vi "sub_DL950_main.vi"(8 "error in":errorcluster) -> (0 "error out":errorcluster, 3 "DL950 wfm":waveform(dbl)[](graph))   [LabVIEW 2019]
uses:
  _ctrl/create-rw-close.ctl
  _ctrl/fgv_DL950.ctl
  _ctrl/rw.ctl
  SubVIs/common/_ctrl/system-status.ctl
  SubVIs/common/Glob_Ref.vi
  Durability/common/Global 1.vi
panel:
  out "items":dbl[][](array[numeric])
  out "Data":string
  out "Waveform":cluster{"l":dbl, "dt":dbl, "Y":dbl[][]}(graph)
  out "n":i32
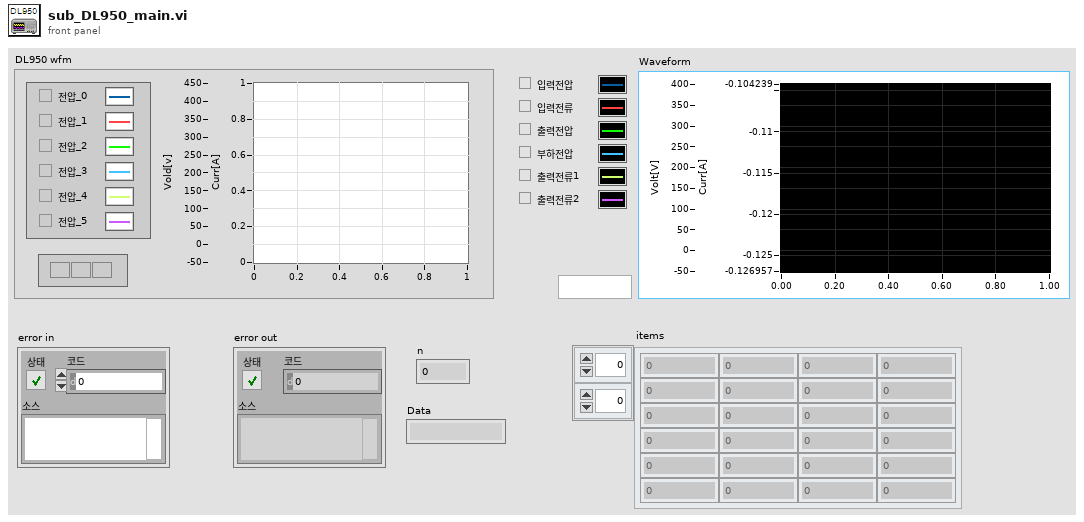
[diagram p1: front panel]
types:
  T1 = typedef "create-rw-close.ctl" = enum16{"create", "write", "read", "delete", "close"}
  T2 = typedef "fgv_DL950.ctl" = enum16{"init", "config", "Set-NCh", "setapply", "trigger", "history_clear", "read", "time-div", "wave-aquis", "start", "query", "abort", "set_items", "reset_items", "read_items", "percent_rise", "trigger_single", "stop", "offset cancel", "close"}
  T3 = typedef "rw.ctl" = enum16{"read", "write"}
  T4 = typedef "system-status.ctl" = enum16{"Initial", "Update", "Clear", "Read"}
  T5 = typedef "start.ctl" = enum16{"init", "open", "set", "start", "stop", "read", "read_items", "query", "close", "T_single", "reset", "exit"}
  T6 = typedef "DL950_wfms.ctl" = cluster{"wfms":waveform(dbl)[], "Waveform_2":cluster{"t0":dbl, "dt":dbl, "Y":dbl[][]}, "items":dbl[][], "da950_array":dbl[]}
  T7 = typedef "ref_all.ctl" = cluster{"BP4610 Config":refnum<vi>, "DSP1950 Config":refnum<vi>, "2470-config":refnum<vi>, "cDAQ 9269 AO config":refnum<vi>, "cDAQ 9221 Config":refnum<vi>, "cDAQ-9467 Config":refnum<vi>, "Waveform":refnum<vi>, "DL950 wfm":refnum<vi>, "AI Graph":refnum<vi>, "AO_Wave-config":refnum<vi>, "DL950 items":refnum<vi>, "Volt":refnum<vi>, "Current":refnum<vi>, "AO_Level":refnum<vi>, "RC-Test Judgement ":refnum<vi>, "Log path":refnum<vi>, "시험명":refnum<vi>, "file renew[Hr]":refnum<vi>, "Breakdown-Spec":refnum<vi>, "paste":refnum<vi>, "copy":refnum<vi>, "DL950_config":refnum<vi>, "종료시간":refnum<vi>, "경과시간":refnum<vi>, "Apply":refnum<vi>, "DSP Config LV ":refnum<vi>, "Testconfig":refnum<vi>}
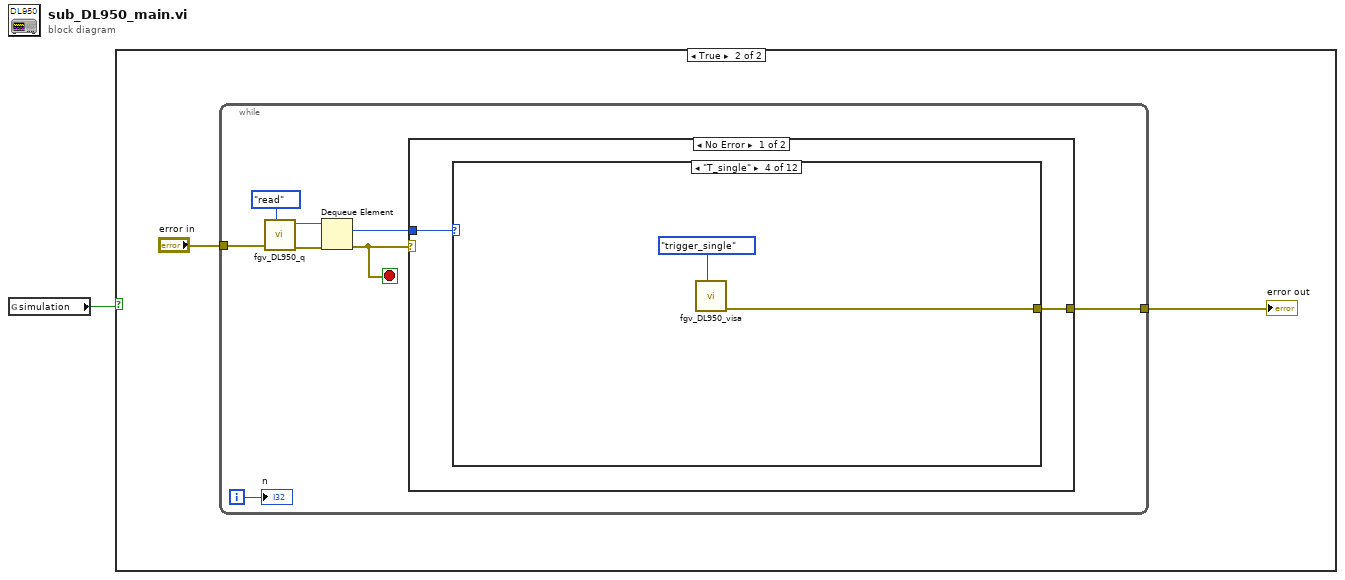
[diagram p0: block diagram]
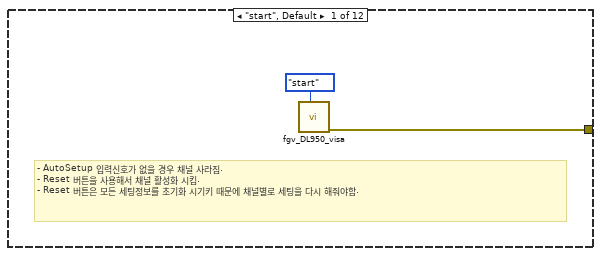
[diagram p3: hidden frame]
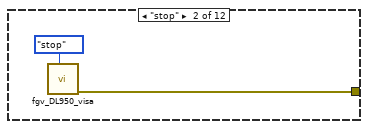
[diagram p4: hidden frame]
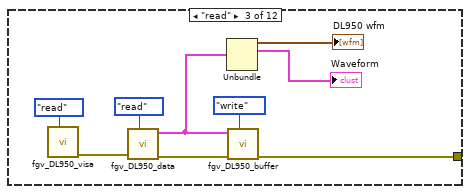
[diagram p5: hidden frame]
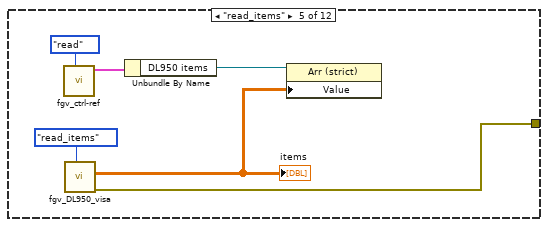
[diagram p6: hidden frame]
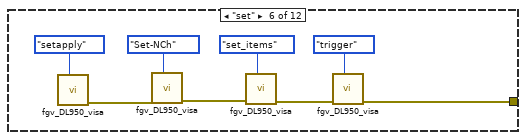
[diagram p7: hidden frame]
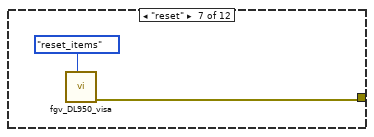
[diagram p8: hidden frame]
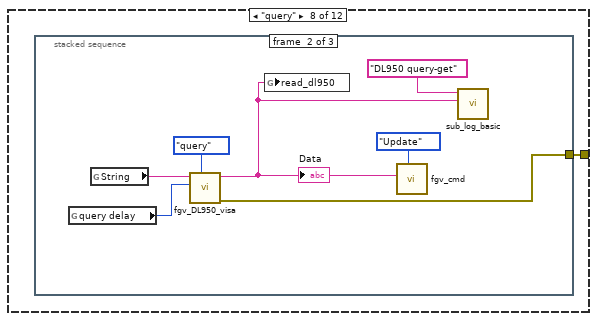
[diagram p9: hidden frame]
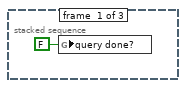
[diagram p10: hidden frame]
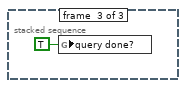
[diagram p11: hidden frame]
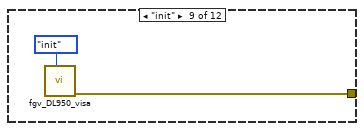
[diagram p12: hidden frame]
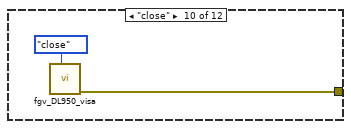
[diagram p13: hidden frame]
diagram:
  n1 = global read "Glob_Ref.vi" "simulation"() -> (w1:bool)
  n2 = case shown="True" w1 {
    frame False {
    }
    frame True {
      n3 = while {
        tunnel: "error in" -> [w5]
        tunnel: [w4] -> w2
        i -> [w7]
        stop <- w6 stop-if-true
        n4 = call "fgv_DL950_q.vi"("cmd"=create-rw-close."read", "error in"=w5) -> ("error out"=w10:errorcluster, "queue out"=w9:refnum<queue>)  [unwired: 8 in]
        n5 = Dequeue Element(queue=w9, error in (no error)=w10) -> (element=w8:T5, error out=w6:errorcluster)  [unwired: 1 in, 2 out]
        n6 = case shown="No Error" w6 {
          selector: w6 -> [_ w59]
          tunnel: w8 -> [w13 _]
          tunnel: [w12 w59] -> w4
          frame No Error {
            n7 = case shown="\"T_single\"" w13 {
              tunnel: [w14 w16 w18 w27 w29 w35 w43 w45 w55 w57 _ _] -> w12
              frame "start", Default {
                # "- AutoSetup 입력신호가 없을 경우 채널 사라짐.\n- Reset 버튼을 사용해서 채널 활성화 시킴.\n- Reset 버튼은 모든 세팅정보를 초기화 시기키 때문에 채널별로 세팅을 다시 해줘야함."
                n8 = call "fgv_DL950_visa.vi"("cmd"=fgv_DL950."start") -> ("error out"=w14:errorcluster)  [unwired: 8 in, 2 out]
              }
              frame "stop" {
                n9 = call "fgv_DL950_visa.vi"("cmd"=fgv_DL950."stop") -> ("error out"=w16:errorcluster)  [unwired: 8 in, 2 out]
              }
              frame "read" {
                n10 = call "fgv_DL950_visa.vi"("cmd"=fgv_DL950."read") -> ("error out"=w23:errorcluster)  [unwired: 8 in, 2 out]
                n11 = call "fgv_DL950_data.vi"("cmd"=rw."read", "error in"=w23) -> ("error out"=w22:errorcluster, "DL950 wfm 2"=w20:T6)  [unwired: 8 in]
                n12 = Unbundle(w20) -> ("wfms"=→"DL950 wfm":waveform(dbl)[], "Waveform_2"=→"Waveform":cluster{"t0":dbl, "dt":dbl, "Y":dbl[][]})  [unwired: 2 out]
                n13 = call "fgv_DL950_buffer.vi"("cmd"=create-rw-close."write", "error in"=w22, "DL950 wfm 2"=w20) -> ("error out"=w18:errorcluster)  [unwired: 7 in, 1 out]
              }
              frame "T_single" {
                n14 = call "fgv_DL950_visa.vi"("cmd"=fgv_DL950."trigger_single") -> ("error out"=w27:errorcluster)  [unwired: 8 in, 2 out]
              }
              frame "read_items" {
                n15 = call "fgv_ctrl-ref.vi"("cmd"=rw."read") -> ("output cluster 2"=w32:T7)  [unwired: 9 in, 1 out]
                n16 = call "fgv_DL950_visa.vi"("cmd"=fgv_DL950."read_items") -> ("error out"=w29:errorcluster, "items"=w30:dbl[][])  [unwired: 8 in, 1 out]
                "items" <- w30
                n17 = Unbundle By Name(w32) -> ("DL950 items"=w31:refnum<vi>)
                n18 = property class="Arr (strict)"(reference=w31, "Value"=w30) -> ()  [unwired: 1 in, 2 out]
              }
              frame "set" {
                n19 = call "fgv_DL950_visa.vi"("cmd"=fgv_DL950."setapply") -> ("error out"=w38:errorcluster)  [unwired: 8 in, 2 out]
                n20 = call "fgv_DL950_visa.vi"("cmd"=fgv_DL950."Set-NCh", "error in"=w38) -> ("error out"=w40:errorcluster)  [unwired: 7 in, 2 out]
                n21 = call "fgv_DL950_visa.vi"("cmd"=fgv_DL950."set_items", "error in"=w40) -> ("error out"=w36:errorcluster)  [unwired: 7 in, 2 out]
                n22 = call "fgv_DL950_visa.vi"("cmd"=fgv_DL950."trigger", "error in"=w36) -> ("error out"=w35:errorcluster)  [unwired: 7 in, 2 out]
              }
              frame "reset" {
                n23 = call "fgv_DL950_visa.vi"("cmd"=fgv_DL950."reset_items") -> ("error out"=w43:errorcluster)  [unwired: 8 in, 2 out]
              }
              frame "query" {
                n24 = stacked-sequence {
                  tunnel: [_ w47 _] -> w45
                  frame #0 {
                    n25 = global write "Global 1.vi" "query done?"(FALSE ("query done?")) -> ()
                  }
                  frame #1 {
                    n26 = global read "Global 1.vi" "query delay"() -> (w50:u32)
                    n27 = global read "Global 1.vi" "String"() -> (w52:string)
                    n28 = call "fgv_DL950_visa.vi"("cmd"=fgv_DL950."query", "ms"=w50, "Initiate"=w52) -> ("error out"=w47:errorcluster, "Data"=w48:string)  [unwired: 6 in, 1 out]
                    "Data" <- w48
                    n29 = global write "Global 1.vi" "read_dl950"(w48) -> ()
                    n30 = call "fgv_cmd.vi"("Mode"=system-status."Update", "Value"=w48) -> ()  [unwired: 9 in, 1 out]
                    n31 = call "sub_log_basic.vi"("desc"=w48, "Title"="DL950 query-get" ("title")) -> ()  [unwired: 9 in, 1 out]
                  }
                  frame #2 {
                    n32 = global write "Global 1.vi" "query done?"(TRUE ("query done?")) -> ()
                  }
                }
              }
              frame "init" {
                n33 = call "fgv_DL950_visa.vi"("cmd"=fgv_DL950."init") -> ("error out"=w55:errorcluster)  [unwired: 8 in, 2 out]
              }
              frame "close" {
                n34 = call "fgv_DL950_visa.vi"("cmd"=fgv_DL950."close") -> ("error out"=w57:errorcluster)  [unwired: 8 in, 2 out]
              }
              frame "exit" {
              }
              frame "open" {
              }
            }
          }
          frame Error {
          }
        }
        "n" <- w7
      }
      "error out" <- w2
    }
  }
